vi "cfg upgrade 2 to 3.vi"(8 "error in":errorcluster, 11 "Engine Configuration In":T2(array[cluster])) -> (0 "error out":errorcluster, 3 "Engine Configuration Out":T3[](array[typedef]))   [LabVIEW 2013, in "Standard Engine Configuration.lvclass"]
uses:
  Standard Engine Configuration.lvclass
  Module Specific Configuration.ctl
  Module Decimation.ctl
  Runtime/error responses.ctl
  error options.ctl
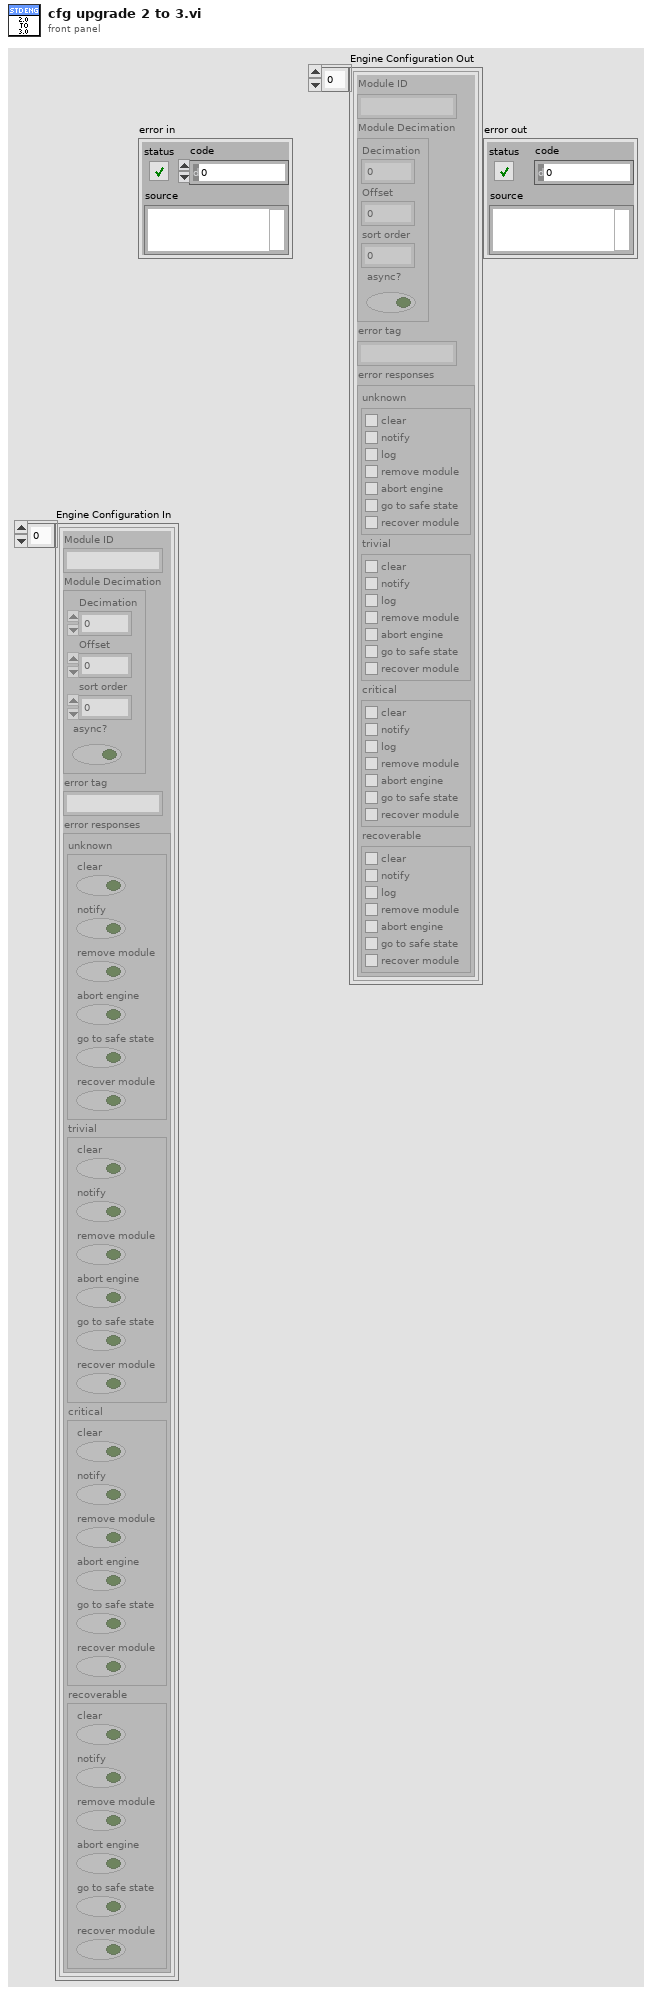
[diagram p1: front panel]
types:
  T1 = typedef "Standard Engine Configuration.lvclass/Module Decimation.ctl" = cluster{"Decimation":u16, "Offset":u16, "sort order":i32, "async?":bool}
  T2 = cluster{"Module ID":string, "Module Decimation":T1, "error tag":string, "error responses":cluster{"unknown":cluster{"clear":bool, "notify":bool, "remove module":bool, "abort engine":bool, "go to safe state":bool, "recover module":bool}, "trivial":cluster{"clear":bool, "notify":bool, "remove module":bool, "abort engine":bool, "go to safe state":bool, "recover module":bool}, "critical":cluster{"clear":bool, "notify":bool, "remove module":bool, "abort engine":bool, "go to safe state":bool, "recover module":bool}, "recoverable":cluster{"clear":bool, "notify":bool, "remove module":bool, "abort engine":bool, "go to safe state":bool, "recover module":bool}}}[]
  T3 = typedef "Standard Engine Configuration.lvclass/Module Specific Configuration.ctl" = cluster{"Module ID":string, "Module Decimation":T1, "error tag":string, "error responses":T4}
  T4 = typedef "Standard Engine Configuration.lvclass/error responses.ctl" = cluster{"unknown":T5, "trivial":T5, "critical":T5, "recoverable":T5}
  T5 = typedef "Standard Engine Configuration.lvclass/error options.ctl" = cluster{"clear":bool, "notify":bool, "log":bool, "remove module":bool, "abort engine":bool, "go to safe state":bool, "recover module":bool}
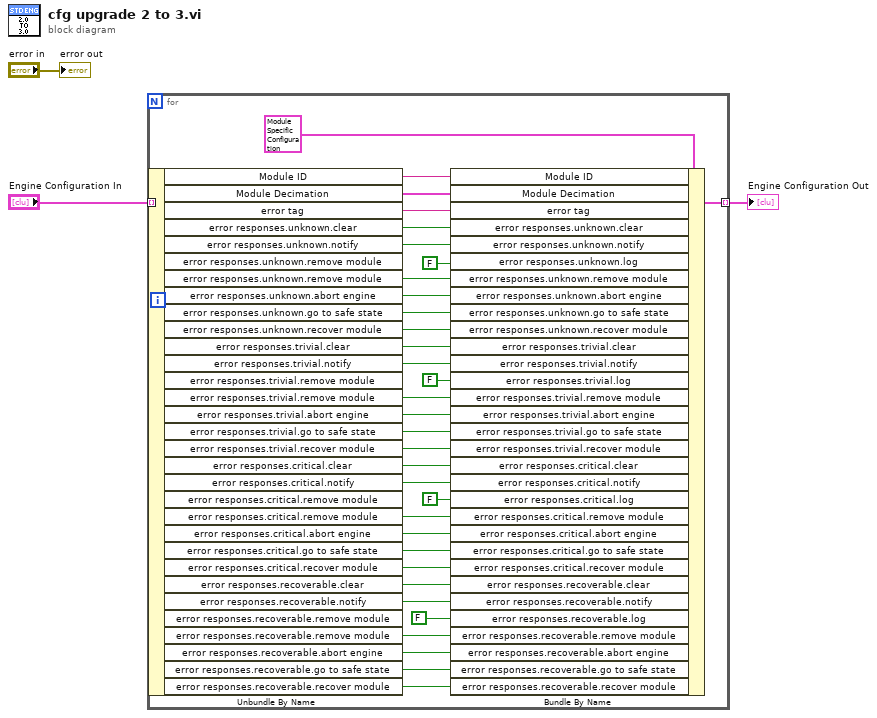
[diagram p0: block diagram]
diagram:
  n1 = for {
    tunnel: "Engine Configuration In" -> [w37] mode=indexing
    tunnel: [w35] -> w1 mode=indexing
    n2 = Unbundle By Name(w37) -> ("Module ID"=w34:string, "Module Decimation"=w33:T1, "error tag"=w32:string, "error responses.unknown.clear"=w31:bool, "error responses.unknown.notify"=w30:bool, "error responses.unknown.remove module"=w25:bool, "error responses.unknown.abort engine"=w26:bool, "error responses.unknown.go to safe state"=w29:bool, "error responses.unknown.recover module"=w28:bool, "error responses.trivial.clear"=w24:bool, "error responses.trivial.notify"=w23:bool, "error responses.trivial.remove module"=w21:bool, "error responses.trivial.abort engine"=w20:bool, "error responses.trivial.go to safe state"=w19:bool, "error responses.trivial.recover module"=w18:bool, "error responses.critical.clear"=w17:bool, "error responses.critical.notify"=w16:bool, "error responses.critical.remove module"=w14:bool, "error responses.critical.abort engine"=w13:bool, "error responses.critical.go to safe state"=w12:bool, "error responses.critical.recover module"=w11:bool, "error responses.recoverable.clear"=w10:bool, "error responses.recoverable.notify"=w9:bool, "error responses.recoverable.remove module"=w7:bool, "error responses.recoverable.abort engine"=w6:bool, "error responses.recoverable.go to safe state"=w5:bool, "error responses.recoverable.recover module"=w4:bool)  [unwired: 4 out]
    n3 = Bundle By Name(cluster=T3 {"Module ID"="", "Module Decimation"={"Decimation"=0, "Offset"=0, "sort order"=0, "async?"=FALSE}, "error tag"="", "error responses"={"unknown"={"clear"=FALSE, "notify"=FALSE, "log"=FALSE, "remove module"=FALSE, "abort engine"=FALSE, "go to safe state"=FALSE, "recover module"=FALSE}, "trivial"={"clear"=FALSE, "notify"=FALSE, "log"=FALSE, "remove module"=FALSE, "abort engine"=FALSE, "go to safe state"=FALSE, "recover module"=FALSE}, "critical"={"clear"=FALSE, "notify"=FALSE, "log"=FALSE, "remove module"=FALSE, "abort engine"=FALSE, "go to safe state"=FALSE, "recover module"=FALSE}, "recoverable"={"clear"=FALSE, "notify"=FALSE, "log"=FALSE, "remove module"=FALSE, "abort engine"=FALSE, "go to safe state"=FALSE, "recover module"=FALSE}}} ("Module Specific Configuration"), "Module ID"=w34, "Module Decimation"=w33, "error tag"=w32, "error responses.unknown.clear"=w31, "error responses.unknown.notify"=w30, "error responses.unknown.log"=FALSE, "error responses.unknown.remove module"=w25, "error responses.unknown.abort engine"=w26, "error responses.unknown.go to safe state"=w29, "error responses.unknown.recover module"=w28, "error responses.trivial.clear"=w24, "error responses.trivial.notify"=w23, "error responses.trivial.log"=FALSE, "error responses.trivial.remove module"=w21, "error responses.trivial.abort engine"=w20, "error responses.trivial.go to safe state"=w19, "error responses.trivial.recover module"=w18, "error responses.critical.clear"=w17, "error responses.critical.notify"=w16, "error responses.critical.log"=FALSE, "error responses.critical.remove module"=w14, "error responses.critical.abort engine"=w13, "error responses.critical.go to safe state"=w12, "error responses.critical.recover module"=w11, "error responses.recoverable.clear"=w10, "error responses.recoverable.notify"=w9, "error responses.recoverable.log"=FALSE, "error responses.recoverable.remove module"=w7, "error responses.recoverable.abort engine"=w6, "error responses.recoverable.go to safe state"=w5, "error responses.recoverable.recover module"=w4) -> (w35:T3)
  }
  "Engine Configuration Out" <- w1
  "error out" <- "error in"
